vi "绘制边框.vi"(4 "填充":bool caption="填充？(F)", 6 "颜色":u32(colorbox) caption="颜色（黑色）", 8 "画笔":T2={"Width"=1, "Style"=enum."Solid"}, 9 "大小":T1 caption="边界", 10 "中心":cluster{"x":i16, "y":i16}, 11 "picture":picture caption="图片") -> (3 "new picture":picture)   [LabVIEW 2018]
uses:
  <vilib>/Utility/miscctls.llb/LVBoundsTypeDef.ctl
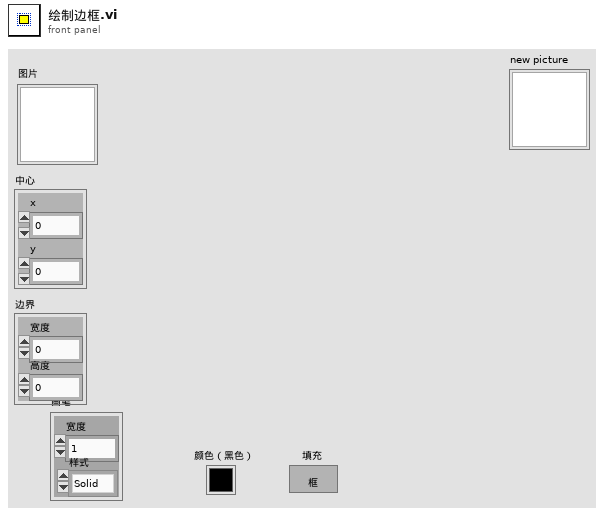
[diagram p1: front panel]
types:
  T1 = typedef "LVBoundsTypeDef.ctl" = cluster{"Width":u32, "Height":u32}
  T2 = cluster{"Width":i16, "Style":enum32{"Solid", "Dash", "Dot", "DashDot", "DashDotDot"}}
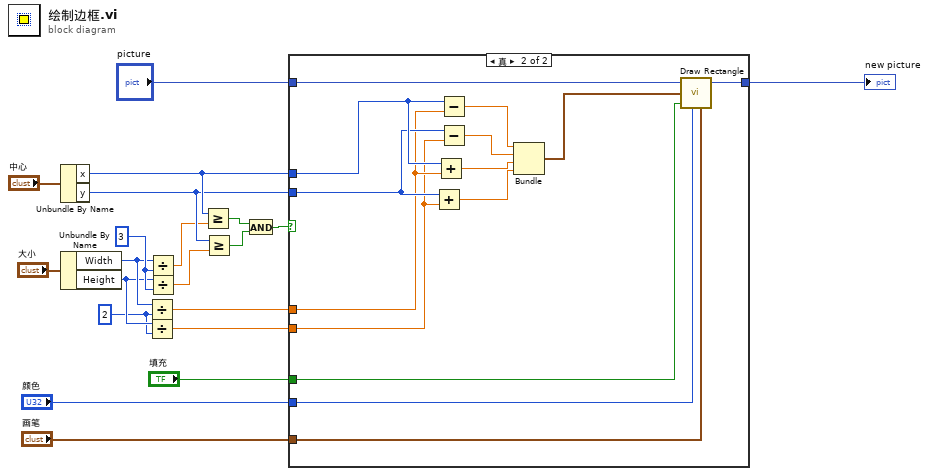
[diagram p0: block diagram]
diagram:
  w3 = u32 2 ("y")
  w6 = u32 3 ("y")
  n1 = Unbundle By Name("中心") -> ("x"=w16:i16, "y"=w15:i16)
  n2 = Unbundle By Name("大小") -> ("Width"=w5:u32, "Height"=w4:u32)
  n3 = Divide(x=w5, y=w3) -> (x/y=w2:dbl)
  n4 = Divide(x=w4, y=w3) -> (x/y=w1:dbl)
  n5 = Divide(x=w5, y=w6) -> (x/y=w8:dbl)
  n6 = Divide(x=w4, y=w6) -> (x/y=w7:dbl)
  n7 = Greater Or Equal?(x=w16, y=w8) -> (x >= y?=w17:bool)
  n8 = Greater Or Equal?(x=w15, y=w7) -> (x >= y?=w14:bool)
  n9 = And(x=w17, y=w14) -> (x .and. y?=w18:bool)
  n10 = case shown="真" w18 {
    tunnel: w16 -> [_ w31]
    tunnel: w15 -> [_ w30]
    tunnel: [w21 w28] -> w10
    tunnel: "picture" -> [w21 w27]
    tunnel: "画笔" -> [_ w26]
    tunnel: "颜色" -> [_ w25]
    tunnel: "填充" -> [_ w24]
    tunnel: w2 -> [_ w23]
    tunnel: w1 -> [_ w22]
    frame False {
    }
    frame True {
      n11 = Add(x=w30, y=w22) -> (x+y=w32:dbl)
      n12 = Add(x=w31, y=w23) -> (x+y=w33:dbl)
      n13 = Subtract(x=w31, y=w23) -> (x-y=w35:dbl)
      n14 = Subtract(x=w30, y=w22) -> (x-y=w34:dbl)
      n15 = Bundle(w35, w34, w33, w32) -> (w29:cluster{dbl, dbl, dbl, dbl})  [unwired: 1 in]
      n16 = call <vilib>:"Draw Rectangle.vi"("picture"=w27, "rect"=w29, "fill?(F)"=w24, "color(black)"=w25, "pen"=w26) -> ("new picture"=w28:picture)  [unwired: 4 in]
    }
  }
  "new picture" <- w10
